vi "2 Trabajo.vi"() -> ()   [LabVIEW 2013]
panel:
  out "Contador":dbl
  out "Numero 50-150":dbl
  # "Generar 10 numeros entre 50-150, usar un ciclo while para validar que el numero se encuentre \nen ese rango antes de presentarlos.  Ir contando los numeros"
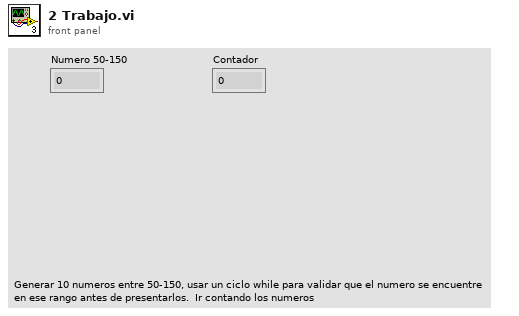
[diagram p1: front panel]
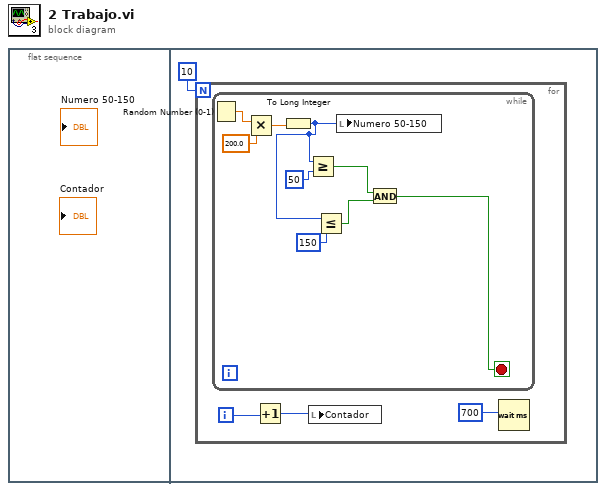
[diagram p0: block diagram]
diagram:
  n1 = flat-sequence {
    frame #0 {
    }
    frame #1 {
      n2 = for {
        N: 10 -> [_]
        i -> [w4]
        n3 = while {
          stop <- w5 stop-if-true
          n4 = Random Number (0-1)() -> (number: 0 to 1=w12:dbl)
          n5 = Multiply(x=w12, y=200.0) -> (x*y=w11:dbl)
          n6 = To Long Integer(number=w11) -> (32bit integer=w8:i32)
          n7 = Greater Or Equal?(x=w8, y=50) -> (x >= y?=w6:bool)
          n8 = Less Or Equal?(x=w8, y=150) -> (x <= y?=w7:bool)
          n9 = local write "Numero 50-150"(w8) -> ()
          n10 = And(x=w6, y=w7) -> (x .and. y?=w5:bool)
        }
        n11 = Increment(x=w4) -> (x+1=w3:i32)
        n12 = local write "Contador"(w3) -> ()
        n13 = Wait (ms)(milliseconds to wait=700) -> ()  [unwired: 1 out]
      }
    }
  }
